vi "Is Dispense Boolean.vi"(8 "error in (no error)":errorcluster, 11 "SecureRelease Syringe in":refnum<class "SecureRelease Syringe.lvclass">) -> (0 "error out":errorcluster, 2 "Is Dispense?":bool, 3 "SecureRelease Syringe out":refnum<class "SecureRelease Syringe.lvclass">)   [LabVIEW 2020, in "SecureRelease Syringe.lvclass"]
uses:
  SecureRelease Syringe.lvclass
  Routine.lvclass
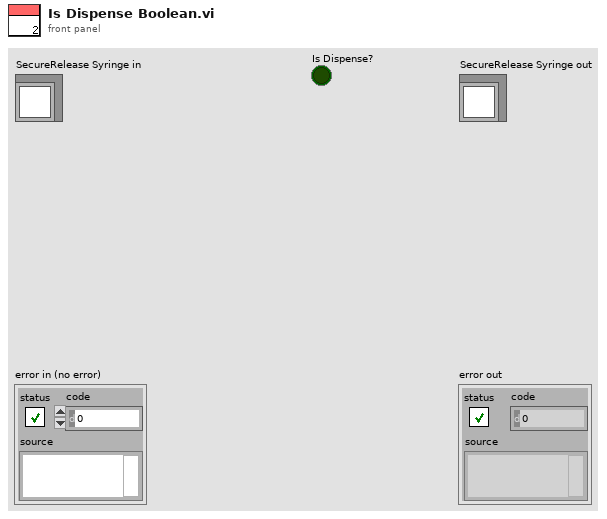
[diagram p1: front panel]
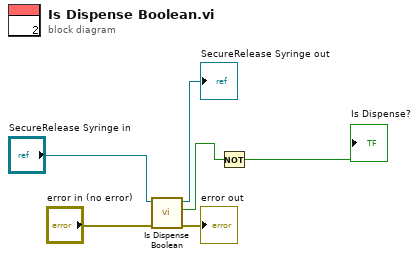
[diagram p0: block diagram]
diagram:
  n1 = call-parent "Is Dispense Boolean.vi"("error in (no error)"="error in (no error)", "Routine in"="SecureRelease Syringe in") -> ("error out"=→"error out":errorcluster, "Is Dispense?"=w2:bool, "Routine out"=→"SecureRelease Syringe out":refnum<class "SecureRelease Syringe.lvclass">)  [unwired: 7 in]
  n2 = Not(x=w2) -> (.not. x?=→"Is Dispense?":bool)
